vi "3 tote hard code.vi"() -> ()   [LabVIEW 2014]
uses:
  Begin/Global Variables.vi
panel:
  in  "Speed (-1 to 1) 3":dbl=0.8 format="%#_13g"
  in  "Direction (0-359) 3":dbl=180.0 format="%#_13g"
  in  "Distance (inches) 3":dbl=50.0 format="%#_13g"
  in  "Speed (-1 to 1) 2":dbl=0.8 format="%#_13g"
  in  "Direction (0-359) 2":dbl=90.0 format="%#_13g"
  in  "Distance (inches) 2":dbl=100.0 format="%#_13g"
  in  "Speed (-1 to 1)":dbl=0.4 format="%#_13g"
  in  "Direction (0-359)":dbl format="%#_13g"
  in  "Distance (inches)":dbl=170.0 format="%#_13g"
  in  "milliseconds to wait 4":u32=1250
  in  "milliseconds to wait 2":u32=1000
  in  "Time 2":dbl=0.75 format="%#_13g"
  in  "milliseconds to wait 3":u32=1500
  in  "Time":dbl=0.5 format="%#_13g"
  in  "milliseconds to wait":u32=1200
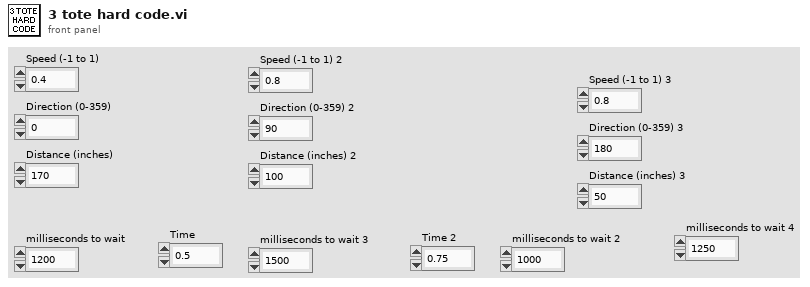
[diagram p1: front panel]
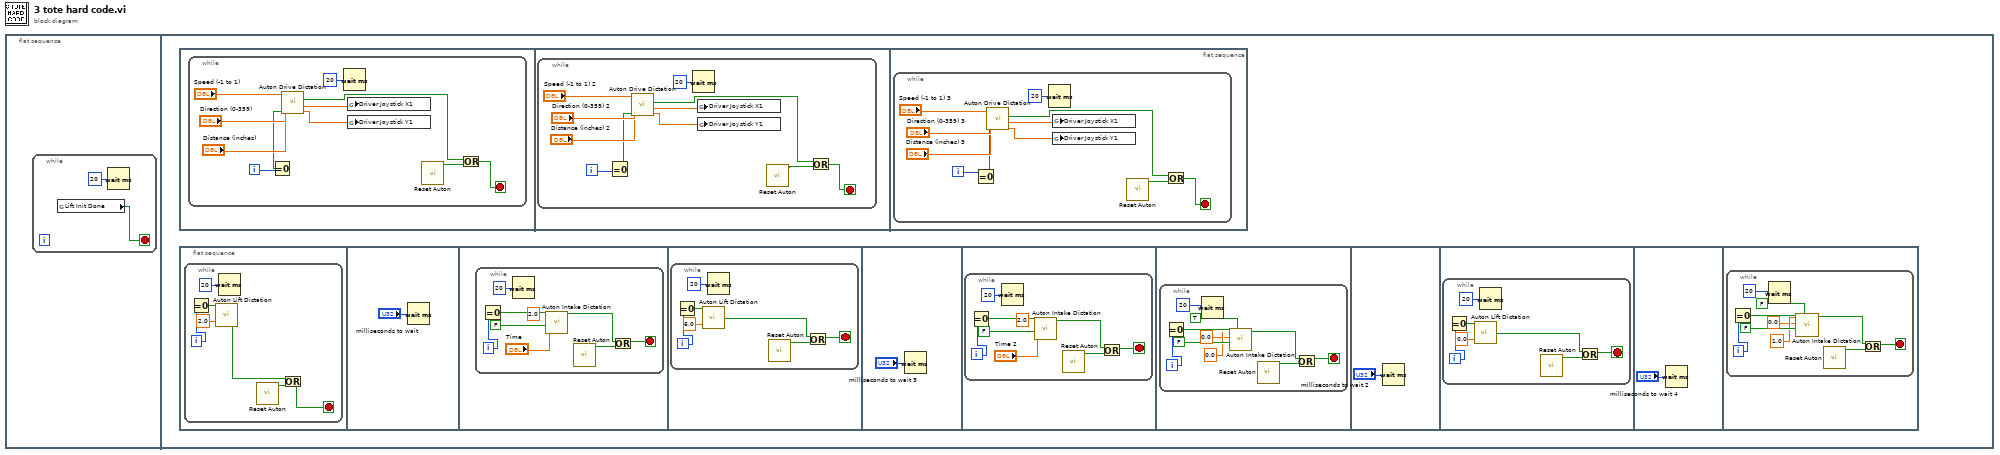
[diagram p0: block diagram]
diagram:
  n1 = flat-sequence {
    frame #0 {
      n2 = while {
        stop <- w2 stop-if-true
        n3 = global read "Global Variables.vi" "Lift Init Done"() -> (w2:bool)
        n4 = Wait (ms)(milliseconds to wait=u32 20) -> ()  [unwired: 1 out]
      }
    }
    frame #1 {
      n5 = flat-sequence {
        frame #0 {
          n6 = while {
            i -> [w8]
            stop <- w3 stop-if-true
            n7 = Equal To 0?(x=w8) -> (x = 0?=w7:bool)
            n8 = call "Auton Lift Dictation.vi"("Level"=2.0, "First Iteration"=w7) -> ("Lift Sequence Done"=w4:bool)
            n9 = Wait (ms)(milliseconds to wait=u32 20) -> ()  [unwired: 1 out]
            n10 = call "Reset Auton.vi"() -> ("Reset Auton"=w5:bool)  [unwired: 11 in]
            n11 = Or(x=w4, y=w5) -> (x .or. y?=w3:bool)
          }
        }
        frame #1 {
          n12 = Wait (ms)(milliseconds to wait="milliseconds to wait") -> ()  [unwired: 1 out]
        }
        frame #2 {
          n13 = while {
            i -> [w19]
            stop <- w14 stop-if-true
            n14 = Equal To 0?(x=w19) -> (x = 0?=w18:bool)
            n15 = Wait (ms)(milliseconds to wait=u32 20) -> ()  [unwired: 1 out]
            n16 = call "Auton Intake Dictation.vi"("First Iteration"=w18, "Roller Arms Same"=FALSE, "Time"="Time", "Intake Select"=2.0) -> ("Time has Elapsed"=w15:bool)  [unwired: 7 in]
            n17 = call "Reset Auton.vi"() -> ("Reset Auton"=w16:bool)  [unwired: 11 in]
            n18 = Or(x=w15, y=w16) -> (x .or. y?=w14:bool)
          }
        }
        frame #3 {
          n19 = while {
            i -> [w25]
            stop <- w20 stop-if-true
            n20 = Equal To 0?(x=w25) -> (x = 0?=w24:bool)
            n21 = call "Auton Lift Dictation.vi"("Level"=6.0, "First Iteration"=w24) -> ("Lift Sequence Done"=w21:bool)
            n22 = Wait (ms)(milliseconds to wait=u32 20) -> ()  [unwired: 1 out]
            n23 = call "Reset Auton.vi"() -> ("Reset Auton"=w22:bool)  [unwired: 11 in]
            n24 = Or(x=w21, y=w22) -> (x .or. y?=w20:bool)
          }
        }
        frame #4 {
          n25 = Wait (ms)(milliseconds to wait="milliseconds to wait 3") -> ()  [unwired: 1 out]
        }
        frame #5 {
          n26 = while {
            i -> [w36]
            stop <- w31 stop-if-true
            n27 = Equal To 0?(x=w36) -> (x = 0?=w35:bool)
            n28 = Wait (ms)(milliseconds to wait=u32 20) -> ()  [unwired: 1 out]
            n29 = call "Auton Intake Dictation.vi"("First Iteration"=w35, "Roller Arms Same"=FALSE, "Time"="Time 2", "Intake Select"=2.0) -> ("Time has Elapsed"=w32:bool)  [unwired: 7 in]
            n30 = call "Reset Auton.vi"() -> ("Reset Auton"=w33:bool)  [unwired: 11 in]
            n31 = Or(x=w32, y=w33) -> (x .or. y?=w31:bool)
          }
        }
        frame #6 {
          n32 = while {
            i -> [w46]
            stop <- w41 stop-if-true
            n33 = Equal To 0?(x=w46) -> (x = 0?=w45:bool)
            n34 = Wait (ms)(milliseconds to wait=u32 20) -> ()  [unwired: 1 out]
            n35 = call "Auton Intake Dictation.vi"("Roller Arms In"=TRUE, "First Iteration"=w45, "Roller Arms Same"=FALSE, "Time"=0.0, "Intake Select"=0.0) -> ("Time has Elapsed"=w42:bool)  [unwired: 6 in]
            n36 = call "Reset Auton.vi"() -> ("Reset Auton"=w43:bool)  [unwired: 11 in]
            n37 = Or(x=w42, y=w43) -> (x .or. y?=w41:bool)
          }
        }
        frame #7 {
          n38 = Wait (ms)(milliseconds to wait="milliseconds to wait 2") -> ()  [unwired: 1 out]
        }
        frame #8 {
          n39 = while {
            i -> [w53]
            stop <- w48 stop-if-true
            n40 = Equal To 0?(x=w53) -> (x = 0?=w52:bool)
            n41 = call "Auton Lift Dictation.vi"("Level"=0.0, "First Iteration"=w52) -> ("Lift Sequence Done"=w49:bool)
            n42 = Wait (ms)(milliseconds to wait=u32 20) -> ()  [unwired: 1 out]
            n43 = call "Reset Auton.vi"() -> ("Reset Auton"=w50:bool)  [unwired: 11 in]
            n44 = Or(x=w49, y=w50) -> (x .or. y?=w48:bool)
          }
        }
        frame #9 {
          n45 = Wait (ms)(milliseconds to wait="milliseconds to wait 4") -> ()  [unwired: 1 out]
        }
        frame #10 {
          n46 = while {
            i -> [w65]
            stop <- w60 stop-if-true
            n47 = Equal To 0?(x=w65) -> (x = 0?=w64:bool)
            n48 = Wait (ms)(milliseconds to wait=u32 20) -> ()  [unwired: 1 out]
            n49 = call "Auton Intake Dictation.vi"("Roller Arms In"=FALSE, "First Iteration"=w64, "Roller Arms Same"=FALSE, "Time"=0.0, "Intake Select"=1.0) -> ("Time has Elapsed"=w61:bool)  [unwired: 6 in]
            n50 = call "Reset Auton.vi"() -> ("Reset Auton"=w62:bool)  [unwired: 11 in]
            n51 = Or(x=w61, y=w62) -> (x .or. y?=w60:bool)
          }
        }
      }
      n52 = flat-sequence {
        frame #0 {
          n53 = while {
            i -> [w73]
            stop <- w67 stop-if-true
            n54 = Equal To 0?(x=w73) -> (x = 0?=w72:bool)
            n55 = call "Auton Drive Dictation.vi"("Reset Encoders"=w72, "Distance (inches)"="Distance (inches)", "Direction (0-359)"="Direction (0-359)", "Speed (-1 to 1)"="Speed (-1 to 1)") -> ("Joy Y"=w70:dbl, "Joy X"=w71:dbl, "Distance Reached?"=w66:bool)  [unwired: 5 in]
            n56 = Wait (ms)(milliseconds to wait=u32 20) -> ()  [unwired: 1 out]
            n57 = global write "Global Variables.vi" "Driver Joystick X1"(w71) -> ()
            n58 = global write "Global Variables.vi" "Driver Joystick Y1"(w70) -> ()
            n59 = call "Reset Auton.vi"() -> ("Reset Auton"=w68:bool)  [unwired: 11 in]
            n60 = Or(x=w66, y=w68) -> (x .or. y?=w67:bool)
          }
        }
        frame #1 {
          n61 = while {
            i -> [w84]
            stop <- w79 stop-if-true
            n62 = Equal To 0?(x=w84) -> (x = 0?=w83:bool)
            n63 = call "Auton Drive Dictation.vi"("Reset Encoders"=w83, "Distance (inches)"="Distance (inches) 2", "Direction (0-359)"="Direction (0-359) 2", "Speed (-1 to 1)"="Speed (-1 to 1) 2") -> ("Joy Y"=w81:dbl, "Joy X"=w82:dbl, "Distance Reached?"=w78:bool)  [unwired: 5 in]
            n64 = Wait (ms)(milliseconds to wait=u32 20) -> ()  [unwired: 1 out]
            n65 = global write "Global Variables.vi" "Driver Joystick X1"(w82) -> ()
            n66 = global write "Global Variables.vi" "Driver Joystick Y1"(w81) -> ()
            n67 = call "Reset Auton.vi"() -> ("Reset Auton"=w77:bool)  [unwired: 11 in]
            n68 = Or(x=w78, y=w77) -> (x .or. y?=w79:bool)
          }
        }
        frame #2 {
          n69 = while {
            i -> [w95]
            stop <- w89 stop-if-true
            n70 = Equal To 0?(x=w95) -> (x = 0?=w94:bool)
            n71 = call "Auton Drive Dictation.vi"("Reset Encoders"=w94, "Distance (inches)"="Distance (inches) 3", "Direction (0-359)"="Direction (0-359) 3", "Speed (-1 to 1)"="Speed (-1 to 1) 3") -> ("Joy Y"=w92:dbl, "Joy X"=w93:dbl, "Distance Reached?"=w88:bool)  [unwired: 5 in]
            n72 = Wait (ms)(milliseconds to wait=u32 20) -> ()  [unwired: 1 out]
            n73 = global write "Global Variables.vi" "Driver Joystick X1"(w93) -> ()
            n74 = global write "Global Variables.vi" "Driver Joystick Y1"(w92) -> ()
            n75 = call "Reset Auton.vi"() -> ("Reset Auton"=w90:bool)  [unwired: 11 in]
            n76 = Or(x=w88, y=w90) -> (x .or. y?=w89:bool)
          }
        }
      }
    }
  }
